vi "Main Engine Host Stream.vi"(8 "error in (no error)":errorcluster, 10 "Host Parameters":T1, 11 "Q Refs":T5) -> (0 "error out":errorcluster, 1 "Exit":bool, 3 "Stream":T6)   [LabVIEW 2019, in "CAN Stream Support Workspace Shared.lvlib"]
uses:
  CAN Stream Support Workspace Shared.lvlib
  Types/Host Stream Data.ctl
  Types/Host Stream Queue Refs.ctl
  Types/Host Stream Queue Type.ctl
  Types/Host Stream Queue Command.ctl
  <vilib>/xnet/xnet.llb/XNET Frame CAN.ctl
  <vilib>/xnet/xnet.llb/XNET Frame Type CAN.ctl
  Types/Host Stream Engine Parameters.ctl
  Addon/Addon Shared/Types/Filter Parameters.ctl
  Addon/Addon Shared/Types/Direction Filter.ctl
  Addon/Addon Shared/Types/Type Filter.ctl
  Types/Host Stream Engine Logging State.ctl
  Types/Host Stream Engine State.ctl
  Process CAN Data.vi
  Process CAN State.vi
  <vilib>/dlg_ctls.llb/Space Constant.vi
  Convert Frame Array to String Array.vi
  <vilib>/Utility/error.llb/Trim Whitespace.vi
  Convert Time to UTC String.vi
  <vilib>/Utility/error.llb/Trim Whitespace One-Sided.vi
  <userlib>/_OpenG.lib/array/array.llb/Sort Array__ogtk.vi
  <userlib>/_OpenG.lib/array/array.llb/Sort 2D Array (String)__ogtk.vi
  <vilib>/Utility/libraryn.llb/Check if File or Folder Exists.vi
  <vilib>/Utility/libraryn.llb/Get File Extension.vi
  Addon/Addon Shared/CAN Stream Support Shared.lvlib
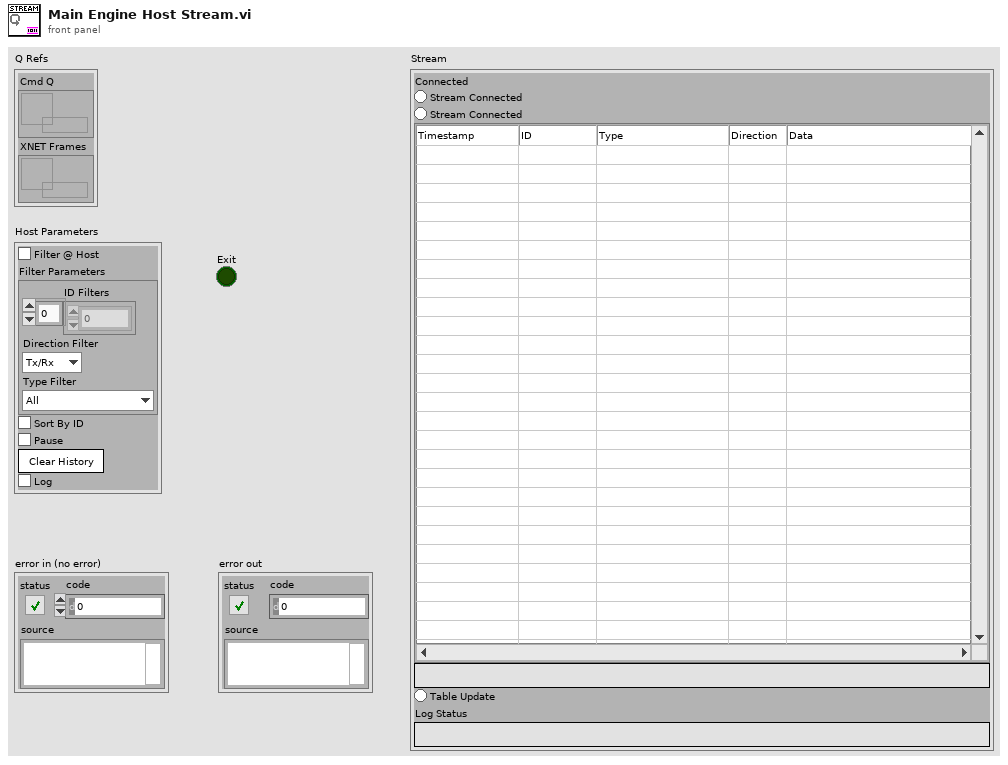
[diagram p1: front panel]
types:
  T1 = typedef "CAN Stream Support Workspace Shared.lvlib/Host Stream Engine Parameters.ctl" = cluster{"Host Filter":bool, "Filter Parameters":T2, "Sort By ID":bool, "Pause":bool, "Clear History":bool, "Log":bool}
  T2 = typedef "CAN Stream Support Shared.lvlib/Filter Parameters.ctl" = cluster{"ID Filters":u32[], "Direction Filter":T3, "Type Filter":T4}
  T3 = typedef "CAN Stream Support Shared.lvlib/Direction Filter.ctl" = enum16{"Tx/Rx", "Rx", "Tx"}
  T4 = typedef "CAN Stream Support Shared.lvlib/Type Filter.ctl" = enum16{"All", "CAN Data", "CAN Remote", "CAN Bus Error", "CAN 2.0 Data", "CAN FD Data", "CAN FD+BRS Data", "J1939 Data", "Delay", "Log Trigger", "Start Trigger"}
  T5 = typedef "CAN Stream Support Workspace Shared.lvlib/Host Stream Queue Refs.ctl" = cluster{"Cmd Q":refnum<queue>, "XNET Frames":refnum<queue>}
  T6 = typedef "CAN Stream Support Workspace Shared.lvlib/Host Stream Data.ctl" = cluster{"Connected":bool, "Bus Data Update":bool, "Bus Data":string[][], "Bus Status":string, "Bus Warning":bool, "Log Status":string}
  T7 = typedef "CAN Stream Support Workspace Shared.lvlib/Host Stream Engine Logging State.ctl" = enum8{"Wait", "Logging", "Cleanup", "Exit"}
  T8 = typedef "CAN Stream Support Workspace Shared.lvlib/Host Stream Engine State.ctl" = enum8{"Wait", "Start Stream", "Read Stream", "Stop Stream", "Exit"}
  T9 = typedef "CAN Stream Support Workspace Shared.lvlib/Host Stream Queue Type.ctl" = cluster{"Cmd":T10, "Target IP Address":string, "Addon":string, "Project Folder":path}
  T10 = typedef "CAN Stream Support Workspace Shared.lvlib/Host Stream Queue Command.ctl" = enum8{"Start Stream", "Stop Stream", "Exit"}
  T11 = typedef "CAN Stream Support Workspace Shared.lvlib/Host Stream Refs.ctl" = cluster{"Target IP Address":string, "Addon":string, "Stream Ref":refnum<k21>}
  T12 = typedef "XNET Frame CAN.ctl" = cluster{"timestamp":timestamp, "payload":u8[], "identifier":u32, "type":T13, "extended?":bool, "echo?":bool}
  T13 = typedef "XNET Frame Type CAN.ctl" = u8
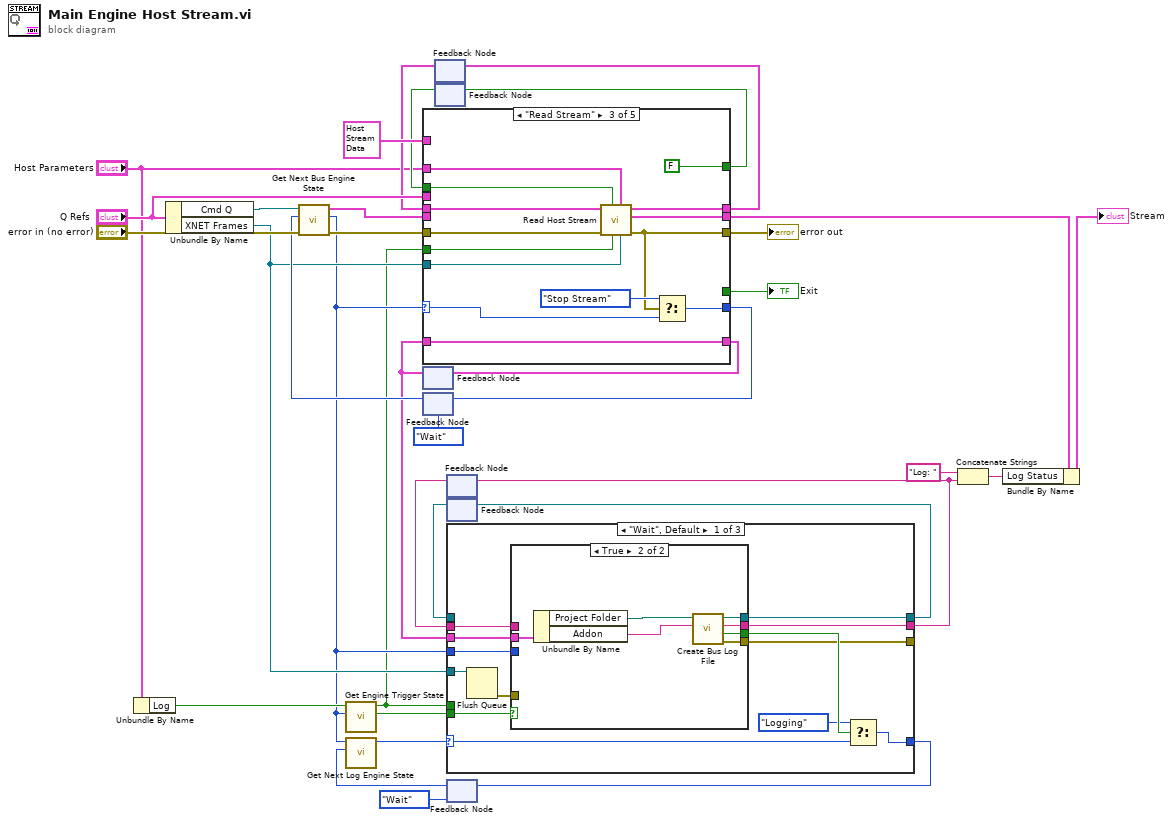
[diagram p0: block diagram]
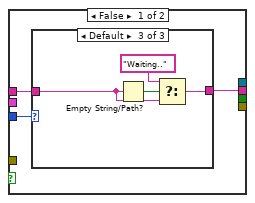
[diagram p2: hidden frame]
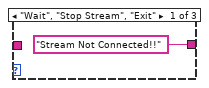
[diagram p3: hidden frame]
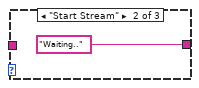
[diagram p4: hidden frame]
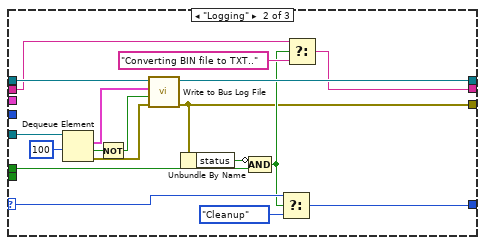
[diagram p5: hidden frame]
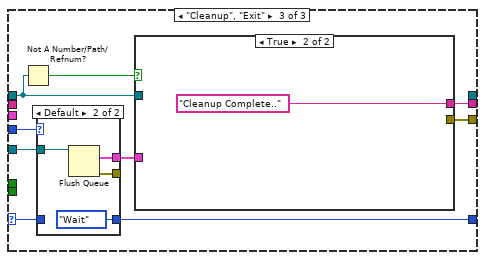
[diagram p6: hidden frame]
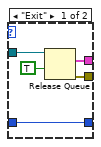
[diagram p7: hidden frame]
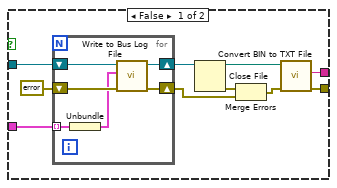
[diagram p8: hidden frame]
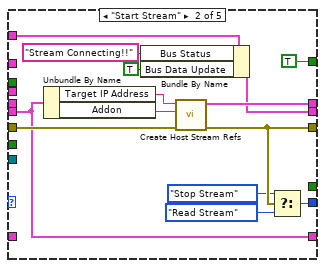
[diagram p10: hidden frame]
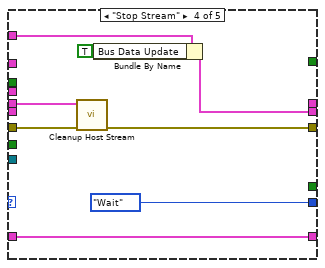
[diagram p11: hidden frame]
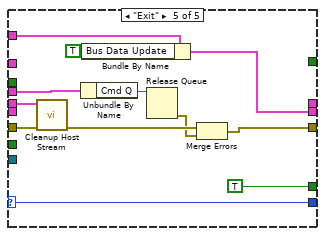
[diagram p12: hidden frame]
diagram:
  n1 = Unbundle By Name("Host Parameters") -> ("Log"=w4:bool)
  n2 = Unbundle By Name("Q Refs") -> ("Cmd Q"=w23:refnum<queue>, "XNET Frames"=w13:refnum<queue>)
  n3 = feedback #1() -> (w8:T9)  [unwired: 1 in]
  n4 = feedback #2(Host_Stream_Engine_State."Wait") -> (w15:T8)
  n5 = call "Get Next Bus Engine State.vi"("error in (no error)"="error in (no error)", "Bus State"=w15, "Cmd Q"=w23) -> ("error out"=w27:errorcluster, "Bus State"=w3:T8, "Command Cluster"=w28:T9)  [unwired: 6 in]
  n6 = call "Get Engine Trigger State.vi"("Bus State"=w3, "Log in"=w4) -> ("Log Trigger"=w2:bool, "Log out"=w1:bool)  [unwired: 8 in]
  n7 = feedback #3() -> (w10:T11)  [unwired: 1 in]
  n8 = feedback #4() -> (w31:bool)  [unwired: 1 in]
  n9 = case shown="\"Read Stream\"" w3 {
    selector: w3 -> [w36 _ w59 _ w83]
    tunnel: w27 -> [w38 w52 w66 w74 w86]
    tunnel: w28 -> [_ w39 _ _ _]
    tunnel: [w38 w48 w60 w73 w75] -> w35
    tunnel: [_ w50 w64 _ _] -> w29
    tunnel: w10 -> [_ _ w65 w72 w85]
    tunnel: [w37 w41 w63 w69 w81] -> w33
    tunnel: [_ TRUE FALSE _ _] -> w30
    tunnel: w31 -> [_ _ w57 _ _]
    tunnel: T6 {"Connected"=FALSE, "Bus Data Update"=FALSE, "Bus Data"=[], "Bus Status"="CAN: Stream Not Connected!!", "Bus Warning"=FALSE, "Log Status"=""} ("Stream") -> [w37 w44 _ w71 w84]
    tunnel: [w36 w45 w58 Host_Stream_Engine_State."Wait" w83] -> w34
    tunnel: [_ _ _ _ TRUE] -> w24
    tunnel: "Q Refs" -> [_ _ _ _ w78]
    tunnel: w13 -> [_ _ w56 _ _]
    tunnel: w1 -> [_ _ w55 _ _]
    tunnel: [_ w39 w54 w67 _] -> w9
    tunnel: w8 -> [_ _ w54 w67 _]
    tunnel: "Host Parameters" -> [_ _ w53 _ _]
    frame "Wait", Default {
    }
    frame "Start Stream" {
      n10 = Unbundle By Name(w39) -> ("Target IP Address"=w51:string, "Addon"=w40:string)
      n11 = Bundle By Name(cluster=w44, "Bus Status"="Stream Connecting!!" ("State"), "Bus Data Update"=TRUE ("Table Update")) -> (w41:T6)
      n12 = call "Create Host Stream Refs.vi"("error in (no error)"=w52, "Addon"=w40, "Target IP Address"=w51) -> ("error out"=w48:errorcluster, "Refs"=w50:T11)  [unwired: 7 in]
      n13 = Select(t=Host_Stream_Engine_State."Stop Stream", s=w48, f=Host_Stream_Engine_State."Read Stream") -> (s? t:f=w45:T8)
    }
    frame "Read Stream" {
      n14 = call "Read Host Stream.vi"("XNET Frames"=w56, "Host Parameters"=w53, "Log"=w55, "Init?"=w57, "error in (no error)"=w66, "Refs in"=w65) -> ("error out"=w60:errorcluster, "Stream"=w63:T6, "Refs out"=w64:T11)  [unwired: 3 in]
      n15 = Select(t=Host_Stream_Engine_State."Stop Stream", s=w60, f=w59) -> (s? t:f=w58:T8)
    }
    frame "Stop Stream" {
      n16 = call "Cleanup Host Stream.vi"("error in (no error)"=w74, "Refs"=w72) -> ("error out"=w73:errorcluster)  [unwired: 9 in]
      n17 = Bundle By Name(cluster=w71, "Bus Data Update"=TRUE ("Table Update")) -> (w69:T6)
    }
    frame "Exit" {
      n18 = call "Cleanup Host Stream.vi"("error in (no error)"=w86, "Refs"=w85) -> ("error out"=w77:errorcluster)  [unwired: 9 in]
      n19 = Unbundle By Name(w78) -> ("Cmd Q"=w79:refnum<queue>)
      n20 = Bundle By Name(cluster=w84, "Bus Data Update"=TRUE ("Table Update")) -> (w81:T6)
      n21 = Release Queue(queue=w79) -> (error out=w76:errorcluster)  [unwired: 2 in, 2 out]
      n22 = Merge Errors(w77, w76) -> (w75:errorcluster)
    }
  }
  "error out" <- w35
  "Exit" <- w24
  n23 = feedback-in #1(w9) -> ()
  n24 = feedback-in #2(w34) -> ()
  n25 = feedback-in #3(w29) -> ()
  n26 = feedback-in #4(w30) -> ()
  n27 = feedback #5() -> (w14:string)  [unwired: 1 in]
  n28 = feedback #6() -> (w17:refnum<file>)  [unwired: 1 in]
  n29 = feedback #7(Host_Stream_Engine_Logging_State."Wait") -> (w20:T7)
  n30 = call "Get Next Log Engine State.vi"("Log State"=w20, "Bus State"=w3) -> ("Log State"=w19:T7)  [unwired: 9 in]
  n31 = case shown="\"Wait\", Default" w19 {
    selector: w19 -> [w97 w126 w136]
    tunnel: w13 -> [w93 w133 w138]
    tunnel: [w99 w128 _] -> w18
    tunnel: w17 -> [_ w129 w141]
    tunnel: [w96 w125 w134] -> w16
    tunnel: w2 -> [w95 _ _]
    tunnel: w1 -> [_ w123 _]
    tunnel: [w94 w118 w140] -> _
    tunnel: [w91 w122 w139] -> w12
    tunnel: w3 -> [w90 _ w137]
    tunnel: w14 -> [w89 w119 _]
    tunnel: w8 -> [w88 _ _]
    frame "Wait", Default {
      n32 = Flush Queue(queue=w93) -> (error out=w92:errorcluster)  [unwired: 1 in, 2 out]
      n33 = case shown="True" w95 {
        tunnel: [_ w115] -> w94
        tunnel: [_ w114] -> w99
        tunnel: [_ w113] -> w98
        tunnel: w92 -> [_ _]
        tunnel: [w101 w112] -> w91
        tunnel: w90 -> [w102 _]
        tunnel: w89 -> [w100 _]
        tunnel: w88 -> [_ w111]
        frame False {
          n34 = case shown="Default" w102 {
            tunnel: ["Stream Not Connected!!" "Waiting.." w106] -> w101
            tunnel: w100 -> [_ _ w105]
            frame "Wait", "Stop Stream", "Exit" {
            }
            frame "Start Stream" {
            }
            frame Default {
              n35 = Empty String/Path?(string/path=w105) -> (empty?=w108:bool)
              n36 = Select(t="Waiting..", s=w108, f=w105) -> (s? t:f=w106:string)
            }
          }
        }
        frame True {
          n37 = Unbundle By Name(w111) -> ("Project Folder"=w110:path, "Addon"=w109:string)
          n38 = call "Create Bus Log File.vi"("Addon"=w109, "Project Folder"=w110) -> ("error out"=w115:errorcluster, "Continue"=w113:bool, "Status"=w112:string, "Byte Stream File out"=w114:refnum<file>)  [unwired: 6 in]
        }
      }
      n39 = Select(t=Host_Stream_Engine_Logging_State."Logging", s=w98, f=w97) -> (s? t:f=w96:T7)
    }
    frame "Logging" {
      n40 = Dequeue Element(queue=w133, timeout in ms (-1)=100) -> (element=w130:T12[], timed out?=w131:bool, error out=w124:errorcluster)  [unwired: 1 in, 1 out]
      n41 = Not(x=w131) -> (.not. x?=w117:bool)
      n42 = call "Write to Bus Log File.vi"("error in (no error)"=w124, "Write?"=w117, "Data"=w130, "Byte Stream File in"=w129) -> ("error out"=w118:errorcluster, "Byte Stream File out"=w128:refnum<file>)  [unwired: 6 in]
      n43 = Unbundle By Name(w118) -> ("status"=w127:bool)
      n44 = Compound Arithmetic op=AND(invert w127, w123) -> (w120:bool)
      n45 = Select(t=w126, s=w120, f=Host_Stream_Engine_Logging_State."Cleanup") -> (s? t:f=w125:T7)
      n46 = Select(t=w119, s=w120, f="Converting BIN file to TXT..") -> (s? t:f=w122:string)
    }
    frame "Cleanup", "Exit" {
      n47 = Not A Number/Path/Refnum?(number/path/refnum=w141) -> (NaN/Path/Refnum?=w142:bool)
      n48 = case shown="Default" w137 {
        tunnel: w138 -> [w147 w151]
        tunnel: [w146 w150] -> w135
        tunnel: [w144 w149] -> _
        tunnel: [w143 Host_Stream_Engine_Logging_State."Wait"] -> w134
        tunnel: w136 -> [w143 _]
        frame "Exit" {
          n49 = Release Queue(queue=w147, force destroy? (F)=TRUE) -> (remaining elements=w146:cluster{"Data":T12[]}[], error out=w144:errorcluster)  [unwired: 1 in, 1 out]
        }
        frame Default {
          n50 = Flush Queue(queue=w151) -> (remaining elements=w150:cluster{"Data":T12[]}[], error out=w149:errorcluster)  [unwired: 1 in, 1 out]
        }
      }
      n51 = case shown="True" w142 {
        tunnel: w141 -> [w161 _]
        tunnel: [w157 _] -> w140
        tunnel: [w153 "Cleanup Complete.."] -> w139
        tunnel: w135 -> [w152 _]
        frame False {
          n52 = for {
            tunnel: w152 -> [w167] mode=indexing
            shift-right: [w165] -> w160
            shift-left: w161 -> [w166]
            shift-right: [w162] -> w156
            shift-left: errorcluster {"status"=FALSE, "code"=0, "source"=""} ("error out") -> [w164]
            n53 = Unbundle(w167) -> ("Data"=w163:T12[])
            n54 = call "Write to Bus Log File.vi"("error in (no error)"=w164, "Data"=w163, "Byte Stream File in"=w166) -> ("error out"=w162:errorcluster, "Byte Stream File out"=w165:refnum<file>)  [unwired: 7 in]
          }
          n55 = Close File(refnum=w160) -> (path=w158:path, error out=w155:errorcluster)  [unwired: 1 in]
          n56 = Merge Errors(w155, w156) -> (w154:errorcluster)
          n57 = call "Convert BIN to TXT File.vi"("error in (no error)"=w154, "path"=w158) -> ("error out"=w157:errorcluster, "Status"=w153:string)  [unwired: 8 in]
        }
        frame True {
        }
      }
    }
  }
  n58 = feedback-in #5(w12) -> ()
  n59 = feedback-in #6(w18) -> ()
  n60 = feedback-in #7(w16) -> ()
  n61 = Concatenate Strings("Log: " ("string"), w12) -> (w5:string)
  n62 = Bundle By Name(cluster=w33, "Log Status"=w5) -> (→"Stream":T6)
